vi "Counter - Single Pulse Output.vi"(6 "Digital Trigger Source":tag="/Dev1/PFI1", 8 "error in":errorcluster, 9 "Pulse Duration":dbl=1e-06 format="%.6f", 10 "Output Terminal":tag="/Dev1/PFI12", 11 "Counter":tag="Dev1/ctr6") -> (0 "error out":errorcluster, 3 "task out":refnum<k21>)   [LabVIEW 2014]
doc: "This example demonstrates how to generate a single pulse using a counter output. \n\nThe single pulse may be triggered once or repeatedly from an external source."
uses:
  <vilib>/DAQmx/create/channels.llb/DAQmx Create Channel (CO-Pulse Generation-Time).vi
  <vilib>/DAQmx/configure/trigger.llb/DAQmx Start Trigger (Digital Edge).vi
  <resource>/objmgr/daqmx.rc
panel:
  in  "Edge":i32(ring)=10280 items=["Rising"=10280, "Falling"=10171]
  # "Channel Settings"
  # "Trigger Settings"
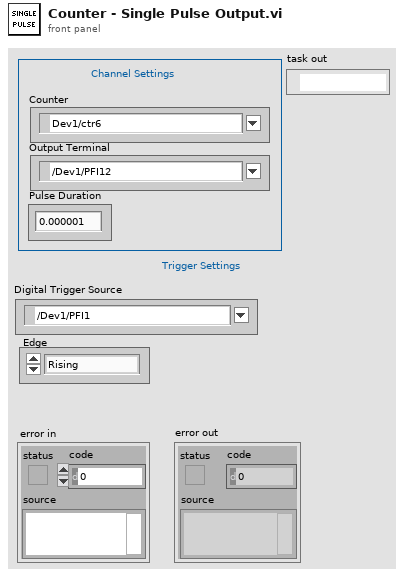
[diagram p1: front panel]
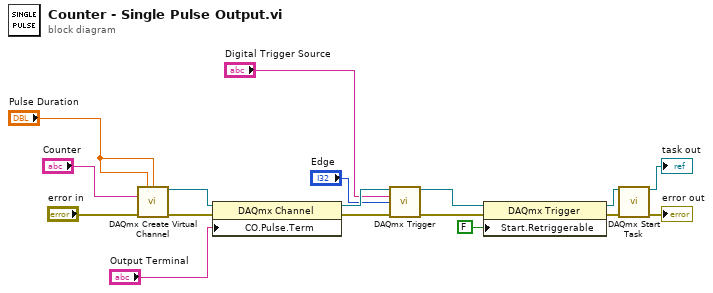
[diagram p0: block diagram]
diagram:
  n1 = call-poly <vilib>:"DAQmx Create Virtual Channel.vi"("high time"="Pulse Duration", "low time"="Pulse Duration", "counter"="Counter", "error in"="error in") -> ("task out"=w14:refnum<k21>, "error out"=w13:errorcluster)  [unwired: 10 in]
  n2 = property class="DAQmx Channel"(reference=w14, error in=w13, "CO.Pulse.Term"="Output Terminal") -> (reference out=w10:refnum<k21>, error out=w11:errorcluster)
  n3 = call-poly <vilib>:"DAQmx Trigger.vi"("task/channels in"=w10, "source"="Digital Trigger Source", "edge"="Edge", "error in"=w11) -> ("task out"=w4:refnum<k21>, "error out"=w5:errorcluster)  [unwired: 10 in]
  n4 = property class="DAQmx Trigger"(reference=w4, error in=w5, "Start.Retriggerable"=FALSE) -> (reference out=w15:refnum<k21>, error out=w16:errorcluster)
  n5 = call <vilib>:"DAQmx Start Task.vi"("task/channels in"=w15, "error in"=w16) -> ("task out"=→"task out":refnum<k21>, "error out"=→"error out":errorcluster)  [unwired: 12 in]
